vi "Connect to SLSC Module and Return Name.vi"(8 "error in (no error)":errorcluster, 10 "connect timeout (4s)":dbl=4.0, 11 "Item Ref Out":T1 format="%.0x") -> (0 "error out":errorcluster, 2 "SLSC Module Name":string, 3 "Item Ref out":T1 format="%.0x")   [LabVIEW 2020, in "SLSC EDS System Explorer.lvlib"]
uses:
  SLSC EDS System Explorer.lvlib
  SLSC CD API/SLSC CD System Explorer/SLSC CD System Explorer.lvlib
  Shared/Constants.vi
  Shared/SLSC EDS Shared.lvlib
  <vilib>/NI VeriStand/Custom Device API/Custom Device Item Ref.ctl
  <vilib>/NI VeriStand/Custom Device API/Custom Device API.lvlib
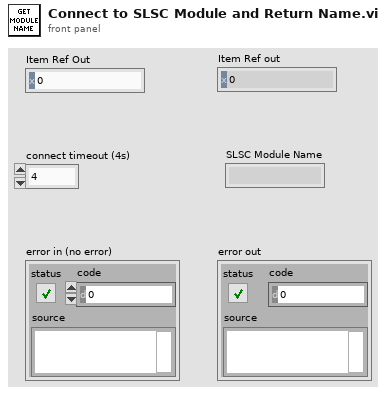
[diagram p1: front panel]
types:
  T1 = typedef "Custom Device API.lvlib/Custom Device Item Ref.ctl" = u64
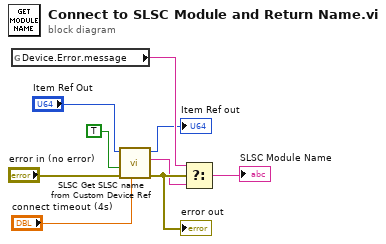
[diagram p0: block diagram]
diagram:
  n1 = global read "Constants.vi" "Device.Error.message"() -> (w3:string)
  n2 = call "SLSC Get SLSC name from Custom Device Ref.vi"("connect timeout"="connect timeout (4s)", "error in (no error)"="error in (no error)", "Wait for mDSN?"=TRUE, "Item Ref in"="Item Ref Out") -> ("error out"=w4:errorcluster, "SLSC Module Name"=w2:string, "Item Ref out"=→"Item Ref out":T1)  [unwired: 4 in, 1 out]
  "error out" <- w4
  n3 = Select(t=w3, s=w4, f=w2) -> (s? t:f=→"SLSC Module Name":string)
